vi "CRYData View Legend Show.vi"(8 "Legend Splitter Position":dbl, 10 "sOption":string, 11 "pGraph VI":refnum<vi>) -> ()   [LabVIEW 2013]
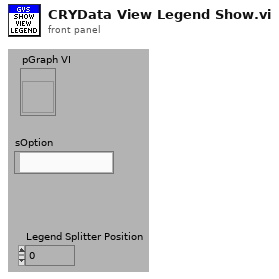
[diagram p1: front panel]
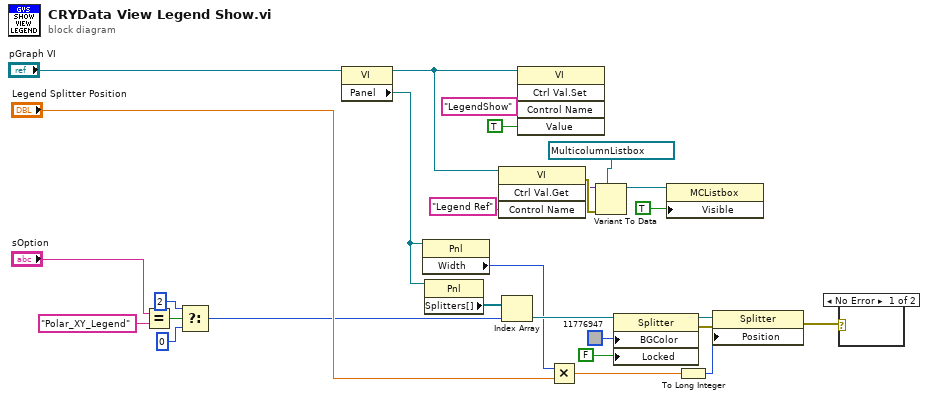
[diagram p0: block diagram]
diagram:
  n1 = Equal?(x="sOption", y="Polar_XY_Legend") -> (x = y?=w24:bool)
  n2 = Select(t=2 ("index"), s=w24, f=0 ("index")) -> (s? t:f=w21:i32)
  n3 = property class="VI"(reference="pGraph VI") -> (reference out=w20:refnum<vi>, "Panel"=w19:refnum<vi>)  [unwired: 1 in, 1 out]
  n4 = property class="Pnl"(reference=w19) -> ("Width"=w5:u32)  [unwired: 1 in, 2 out]
  n5 = property class="Pnl"(reference=w19) -> ("Splitters[]"=w10:refnum<vi>[])  [unwired: 1 in, 2 out]
  n6 = invoke class="VI" method="Ctrl Val.Get"(reference=w20, "Control Name"="Legend Ref") -> (error out=w16:errorcluster, "Get Control Value Variant"=w15:variant)  [unwired: 2 in, 2 out]
  n7 = Index Array(array=w10, index=w21) -> (element=w9:refnum<vi>)
  n8 = invoke class="VI" method="Ctrl Val.Set"(reference=w20, "Control Name"="LegendShow", "Value"=TRUE ("Visible")) -> ()  [unwired: 2 in, 5 out]
  n9 = Multiply(x=w5, y="Legend Splitter Position") -> (x*y=w4:dbl)
  n10 = Variant To Data(error in=w16, type=refnum<vi> refnum ("Legend Ref"), Variant=w15) -> (data=w11:refnum<vi>)  [unwired: 1 out]
  n11 = property on="Property Node" class="Splitter"(reference=w9, "BGColor"=u32 11776947, "Locked"=FALSE ("Splitter Position Locked")) -> (reference out=w6:refnum<vi>, error out=w1:errorcluster)  [unwired: 1 in]
  n12 = property class="MCListbox"(reference=w11, "Visible"=TRUE) -> ()  [unwired: 1 in, 2 out]
  n13 = To Long Integer(number=w4) -> (32bit integer=w3:i32)
  n14 = property on="Property Node" class="Splitter"(reference=w6, error in=w1, "Position"=w3) -> (error out=w2:errorcluster)  [unwired: 1 out]
  n15 = case shown="No Error" w2 {
    frame No Error {
    }
    frame Error {
    }
  }
